vi "TDMS Advanced - Read Synchronously.vi"() -> ()   [LabVIEW 2020]
panel:
  out "Waveform Graph":u32[](graph)
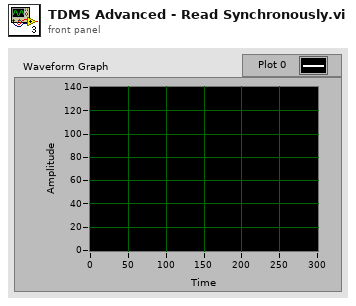
[diagram p1: front panel]
types:
  T1 = enum16{"open", "open or create", "create or replace", "create", "open (read-only)"}
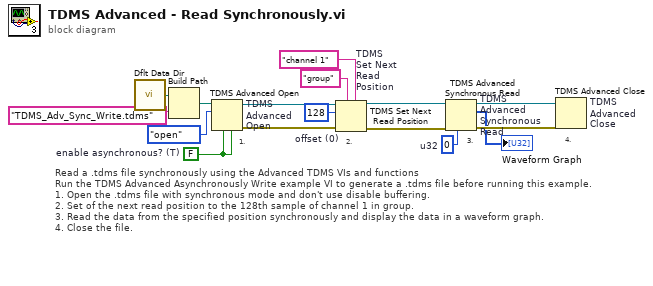
[diagram p0: block diagram]
diagram:
  w5 = i64 128  # offset (0)
  w12 = FALSE  # enable asynchronous? (T)
  w4 = u32 0  # u32
  # "Read a .tdms file synchronously using the Advanced TDMS VIs and functions\nRun the TDMS Advanced Asynchronously Write example VI to generate a .tdms file before running this example.\n1. Open the .tdms file with synchronous mode and don't use disable buffering.\n2. Set of the next read position to the 128th sample of channel 1 in group.\n3. Read the data from the specified position synchronously and display the data in a waveform graph.\n4. Close the file."
  # "1."
  # "4."
  # "3."
  # "2."
  n1 = call <vilib>:"Dflt Data Dir.vi"() -> ("App:Default Data Directory"=w13:path)
  n2 = Build Path(base path=w13, name or relative path="TDMS_Adv_Sync_Write.tdms") -> (appended path=w15:path)
  n3 = TDMS Advanced Open "TDMS\nAdvanced\nOpen"(4:w12, 6:w12, 10:T1."open" ("operation (0:open)"), 11:w15) -> (0:w6:errorcluster, 3:w7:refnum<k34>)  [unwired: 1 in, 1 out]
  n4 = TDMS Set Next Read Position "TDMS\nSet Next\nRead\nPosition"(5:"channel 1", 7:"group" ("group name (Untitled)"), 8:w6, 10:w5, 11:w7) -> (0:w9:errorcluster, 3:w8:refnum<k34>)  [unwired: 1 in]
  n5 = TDMS Advanced Synchronous Read "TDMS\nAdvanced\nSynchronous\nRead"(6:w4, 8:w9, 11:w8) -> (0:w11:errorcluster, 2:→"Waveform Graph":u32[], 3:w10:refnum<k34>)  [unwired: 1 in, 1 out]
  n6 = TDMS Advanced Close "TDMS\nAdvanced\nClose"(8:w11, 11:w10) -> ()  [unwired: 2 in, 2 out]
